vi "Xbox One Controller - Event Based Read.vi"() -> ()   [LabVIEW 2011, in "LVH-Xbox-One-Controller.lvlib"]
doc: "This example demonstrates how to read button and axis data from an Xbox One controller using events."
uses:
  vi.lib/LabVIEW Hacker/Xbox-One-Controller/LVH-Xbox-One-Controller.lvlib
  vi.lib/LabVIEW Hacker/Xbox-One-Controller/Private/Type Defs/Indicators/All Axis Data.ctl
  vi.lib/LabVIEW Hacker/Xbox-One-Controller/Private/Type Defs/Indicators/DPad Enum.ctl
panel:
  in  "Device Index":i32
  out "Event Log":string[](array[string])
  out "All Axis":T1
  in  "Stop Button":bool
  # "Xbox One Controller  - Event Based Read\n\nThis example demonstrates how to read all buttons and axis data from an Xbox One controller using events.\n\nInstructions\n1. Select the Device Index associated with the Xbox One Controller.\n     Note: Use the 'Xbox One Controller - Find Controllers' Example in the LabVIEW Example Finder to determine the device index.\n2. Click the Run Arrow.\n3. Notice the controller Icon on the front panel update to match the actual controller state."
  # "Configure"
  # "Controller Data"
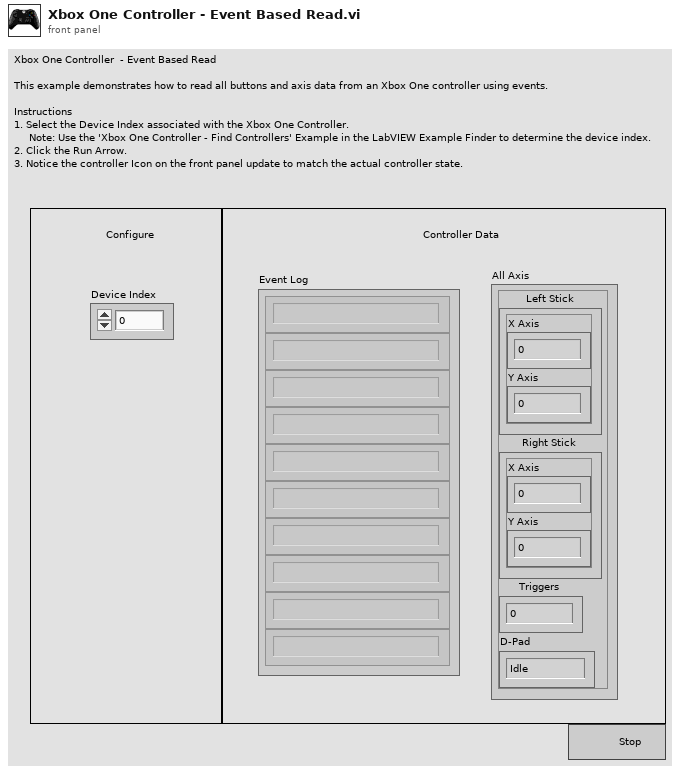
[diagram p1: front panel]
types:
  T1 = typedef "LVH-Xbox-One-Controller.lvlib/All Axis Data.ctl" = cluster{"Left Stick":cluster{"X Axis":i32, "Y Axis":i32}, "Right Stick":cluster{"X Axis":i32, "Y Axis":i32}, "Triggers":i32, "D-Pad":T2}
  T2 = typedef "LVH-Xbox-One-Controller.lvlib/DPad Enum.ctl" = enum16{"Idle", "Up", "Up / Right", "Right", "Down / Right", "Down", "Down / Left", "Left", "Up / Left"}
  T3 = typedef "LVH-Xbox-One-Controller.lvlib/Xbox One Controller Ref.ctl" = cluster{"Controller Ref":refnum<k1>, "Event Refnum":refnum<event-registration>, "Worker Ref":refnum<vi>}
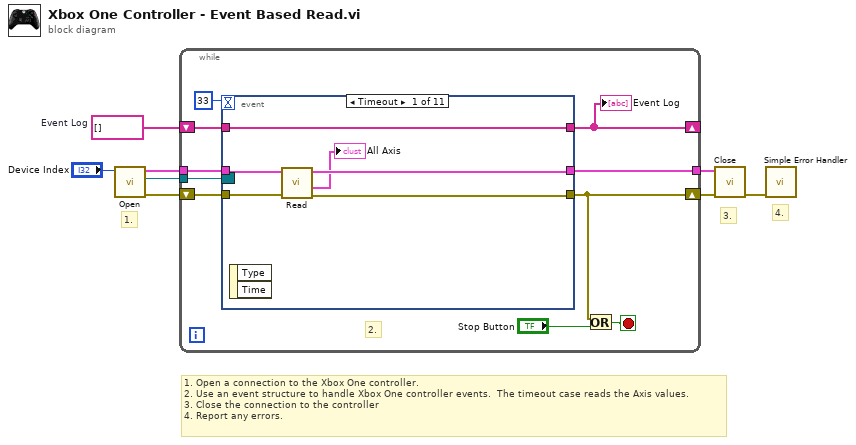
[diagram p0: block diagram]
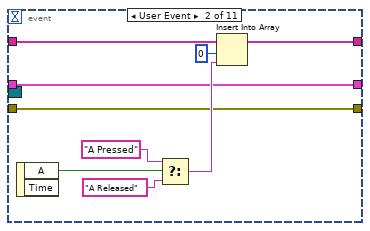
[diagram p2: hidden frame]
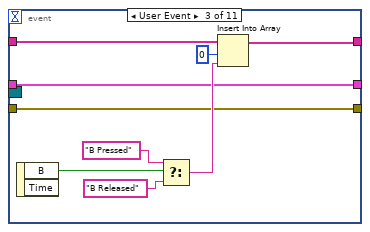
[diagram p3: hidden frame]
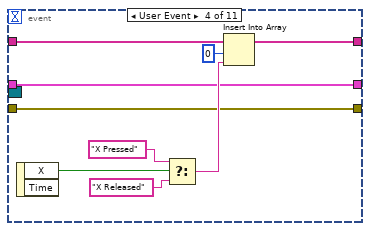
[diagram p4: hidden frame]
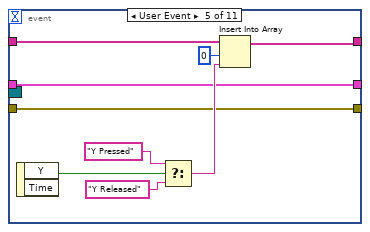
[diagram p5: hidden frame]
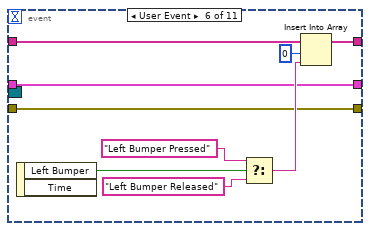
[diagram p6: hidden frame]
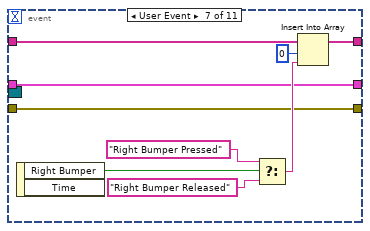
[diagram p7: hidden frame]
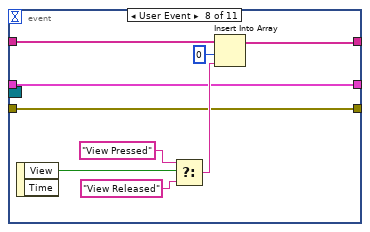
[diagram p8: hidden frame]
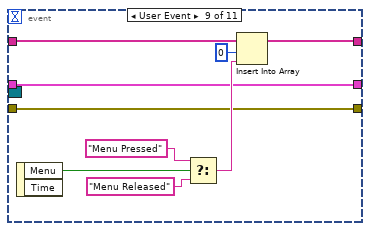
[diagram p9: hidden frame]
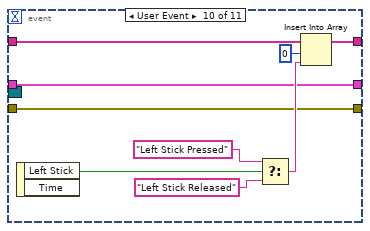
[diagram p10: hidden frame]
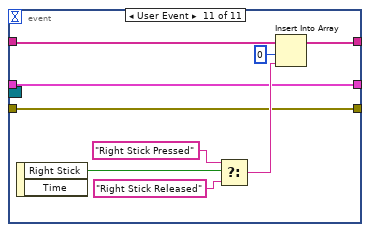
[diagram p11: hidden frame]
diagram:
  w3 = string[] []  # Event Log
  # "1. Open a connection to the Xbox One controller.\n2. Use an event structure to handle Xbox One controller events.  The timeout case reads the Axis values.\n3. Close the connection to the controller\n4. Report any errors."
  # "4."
  # "3."
  # "1."
  n1 = call "Open.vi"("Device Index"="Device Index") -> ("Error Out"=w6:errorcluster, "Event Refnum"=w5:refnum<event-registration>, "Xbox One Controller Ref"=w4:T3)  [unwired: 8 in]
  n2 = while {
    tunnel: w5 -> [w11]
    shift-right: [w14] -> w7
    shift-left: w6 -> [w17]
    tunnel: w4 -> [w18]
    tunnel: [w13] -> w8
    shift-right: [w9] -> _
    shift-left: w3 -> [w10]
    stop <- w16 stop-if-true
    # "2."
    n3 = event shown="[0] Timeout" {
      selector: w11 -> [_ _ _ _ _ _ _ _ _ _ _]
      dyn-events: _ -> [_ _ _ _ _ _ _ _ _ _ _]
      timeout: 33 -> [_ _ _ _ _ _ _ _ _ _ _]
      tunnel: w18 -> [w24 w27 w35 w47 w57 w65 w72 w82 w89 w99 w109]
      tunnel: w17 -> [w23 w26 w36 w48 w56 w66 w73 w83 w90 w98 w108]
      tunnel: [w19 w26 w36 w48 w56 w66 w73 w83 w90 w98 w108] -> w14
      tunnel: [w22 w27 w35 w47 w57 w65 w72 w82 w89 w99 w109] -> w13
      tunnel: w10 -> [w20 w33 w38 w46 w54 w64 w74 w81 w92 w101 w110]
      tunnel: [w20 w28 w37 w45 w53 w63 w75 w80 w93 w102 w111] -> w9
      event Timeout {
        n4 = event-data() -> ()  [unwired: 1 in, 2 out]
        n5 = call "Read.vi"("Error In"=w23, "Xbox One Controller Ref"=w24) -> ("Error Out"=w19:errorcluster, "All Axis"=→"All Axis":T1, "Xbox One Controller Ref"=w22:T3)  [unwired: 6 in, 1 out]
      }
      event User Event {
        n6 = event-data() -> ("A"=w32:bool)  [unwired: 1 in, 1 out]
        n7 = Select(t="A Pressed" ("String"), s=w32, f="A Released" ("String")) -> (s? t:f=w29:string)
        n8 = Insert Into Array(array=w33, index=0, new element=w29) -> (w28:string[])
      }
      event User Event {
        n9 = event-data() -> ("B"=w39:bool)  [unwired: 1 in, 1 out]
        n10 = Select(t="B Pressed" ("String"), s=w39, f="B Released" ("String")) -> (s? t:f=w40:string)
        n11 = Insert Into Array(array=w38, index=0, new element=w40) -> (w37:string[])
      }
      event User Event {
        n12 = event-data() -> ("X"=w44:bool)  [unwired: 1 in, 1 out]
        n13 = Select(t="X Pressed" ("String"), s=w44, f="X Released" ("String")) -> (s? t:f=w49:string)
        n14 = Insert Into Array(array=w46, index=0, new element=w49) -> (w45:string[])
      }
      event User Event {
        n15 = event-data() -> ("Y"=w55:bool)  [unwired: 1 in, 1 out]
        n16 = Select(t="Y Pressed" ("String"), s=w55, f="Y Released" ("String")) -> (s? t:f=w58:string)
        n17 = Insert Into Array(array=w54, index=0, new element=w58) -> (w53:string[])
      }
      event User Event {
        n18 = event-data() -> ("Left Bumper"=w62:bool)  [unwired: 1 in, 1 out]
        n19 = Select(t="Left Bumper Pressed" ("String"), s=w62, f="Left Bumper Released" ("String")) -> (s? t:f=w67:string)
        n20 = Insert Into Array(array=w64, index=0, new element=w67) -> (w63:string[])
      }
      event User Event {
        n21 = event-data() -> ("Right Bumper"=w71:bool)  [unwired: 1 in, 1 out]
        n22 = Select(t="Right Bumper Pressed" ("String"), s=w71, f="Right Bumper Released" ("String")) -> (s? t:f=w76:string)
        n23 = Insert Into Array(array=w74, index=0, new element=w76) -> (w75:string[])
      }
      event User Event {
        n24 = event-data() -> ("View"=w84:bool)  [unwired: 1 in, 1 out]
        n25 = Select(t="View Pressed" ("String"), s=w84, f="View Released" ("String")) -> (s? t:f=w85:string)
        n26 = Insert Into Array(array=w81, index=0, new element=w85) -> (w80:string[])
      }
      event User Event {
        n27 = event-data() -> ("Menu"=w91:bool)  [unwired: 1 in, 1 out]
        n28 = Select(t="Menu Pressed" ("String"), s=w91, f="Menu Released" ("String")) -> (s? t:f=w94:string)
        n29 = Insert Into Array(array=w92, index=0, new element=w94) -> (w93:string[])
      }
      event User Event {
        n30 = event-data() -> ("Left Stick"=w100:bool)  [unwired: 1 in, 1 out]
        n31 = Select(t="Left Stick Pressed" ("String"), s=w100, f="Left Stick Released" ("String")) -> (s? t:f=w103:string)
        n32 = Insert Into Array(array=w101, index=0, new element=w103) -> (w102:string[])
      }
      event User Event {
        n33 = event-data() -> ("Right Stick"=w107:bool)  [unwired: 1 in, 1 out]
        n34 = Select(t="Right Stick Pressed" ("String"), s=w107, f="Right Stick Released" ("String")) -> (s? t:f=w112:string)
        n35 = Insert Into Array(array=w110, index=0, new element=w112) -> (w111:string[])
      }
    }
    "Event Log" <- w9
    n36 = Or(x=w14, y="Stop Button") -> (x .or. y?=w16:bool)
  }
  n37 = call "Close.vi"("Error In"=w7, "Xbox One Controller Ref"=w8) -> ("Error Out"=w1:errorcluster)  [unwired: 9 in]
  n38 = call <vilib>:"Simple Error Handler.vi"("error in (no error)"=w1) -> ()  [unwired: 4 in, 5 out]
